vi "HTML_ArrayToAttributeString.vi"(10 "Attribute List[]":string[](array[string])) -> (2 "spreadsheet string":string)   [LabVIEW 2014]
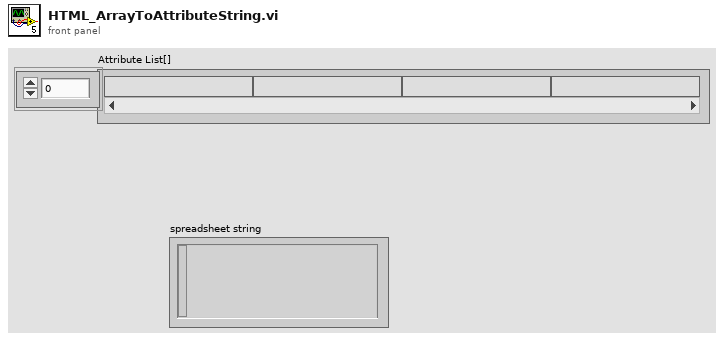
[diagram p1: front panel]
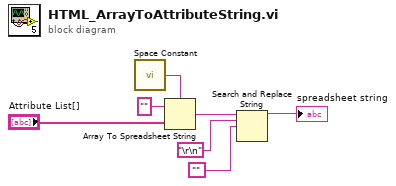
[diagram p0: block diagram]
diagram:
  n1 = call <vilib>:"Space Constant.vi"() -> ("String"=w6:string)
  n2 = Array To Spreadsheet String(delimiter (Tab)=w6, array="Attribute List[]", 3:"" ("format string")) -> (spreadsheet string=w4:string)
  n3 = Search and Replace String(input string=w4, search string="\r\n", replace string="") -> (result string=→"spreadsheet string":string)  [unwired: 5 in, 3 out]
